vi "get_version.vi"(8 "error in (no error)":errorcluster) -> (0 "error out":errorcluster, 2 "Bus version":string, 3 "DLL version":string)   [LabVIEW 2014, in "Dali_usb.lvlib"]
uses:
  Dali_usb.lvlib
  dll/DaliBusAccess.dll
  Deploy/Utilities/Miscelanous.lvlibp
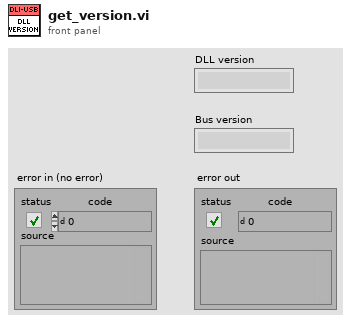
[diagram p1: front panel]
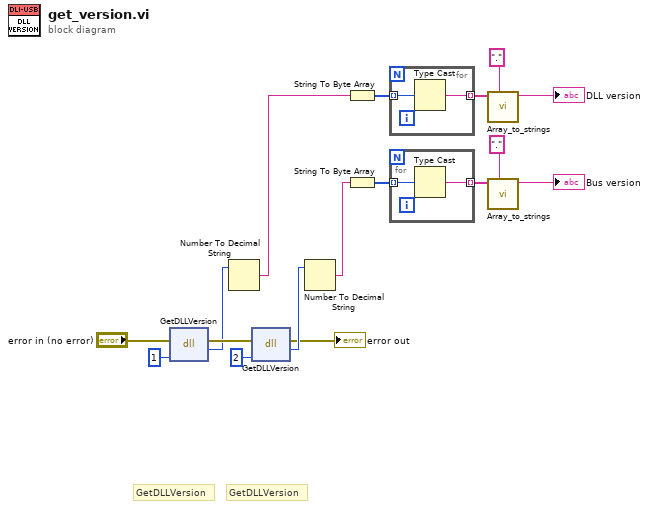
[diagram p0: block diagram]
diagram:
  # "GetDLLVersion"
  # "GetDLLVersion"
  n1 = dll-call lib="C:/LTS/app-tde-luminaires/SourceCode/Instruments/Driver_interaction/Dali_usb/Vendor/dll/DaliBusAccess.dll" fn="GetDLLVersion"(error in="error in (no error)", "iIndex"=1) -> (error out=w14:errorcluster, "return type"=w13:i32)  [unwired: 3 in, 1 out]
  n2 = Number To Decimal String(number=w13) -> (decimal integer string=w12:string)  [unwired: 1 in]
  n3 = dll-call lib="C:/LTS/app-tde-luminaires/SourceCode/Instruments/Driver_interaction/Dali_usb/Vendor/dll/DaliBusAccess.dll" fn="GetDLLVersion"(error in=w14, "iIndex"=2) -> (error out=→"error out":errorcluster, "return type"=w17:i32)  [unwired: 3 in, 1 out]
  n4 = Number To Decimal String(number=w17) -> (decimal integer string=w3:string)  [unwired: 1 in]
  n5 = String To Byte Array(string=w12) -> (unsigned byte array=w11:u8[])
  n6 = String To Byte Array(string=w3) -> (unsigned byte array=w5:u8[])
  n7 = for {
    tunnel: w11 -> [w19] mode=indexing
    tunnel: [w18] -> w10 mode=indexing
    n8 = Type Cast(x=w19) -> (*(type *) &x=w18:string)  [unwired: 1 in]
  }
  n9 = for {
    tunnel: w5 -> [w21] mode=indexing
    tunnel: [w20] -> w6 mode=indexing
    n10 = Type Cast(x=w21) -> (*(type *) &x=w20:string)  [unwired: 1 in]
  }
  n11 = call "Array_to_strings.vi"("delimeter (;)"=".", "Array of strings"=w10) -> ("delimited string"=→"DLL version":string)  [unwired: 9 in]
  n12 = call "Array_to_strings.vi"("delimeter (;)"=".", "Array of strings"=w6) -> ("delimited string"=→"Bus version":string)  [unwired: 9 in]
